vi "table_doubling.vi"() -> ()   [LabVIEW 2014]
panel:
  in  "append_element":dbl format="%#_13g"
  in  "input_arr":dbl[](array[numeric])
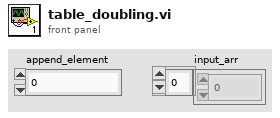
[diagram p1: front panel]
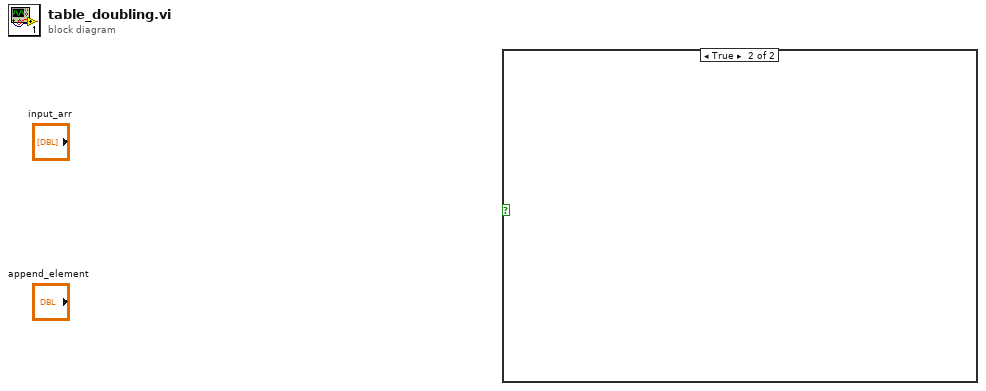
[diagram p0: block diagram]
diagram:
  n1 = case shown="True" {
    selector: _ -> [_ _]
    frame False {
    }
    frame True {
    }
  }
